vi "DSF.Engine.BuilderManager.Builder FIFO.Write.vi"(8 "error in (no error)":errorcluster, 9 "timeout in ms (0)":i32, 10 "Builder ID":i32, 11 "Builder Manager in":refnum<class "DSF.Engine.BuilderManager.lvclass">) -> (0 "error out":errorcluster, 1 "timed out?":bool, 3 "Builder Manager out":refnum<class "DSF.Engine.BuilderManager.lvclass">)   [LabVIEW 2016, in "DSF.Engine.lvlib" / "DSF.Engine.BuilderManager.lvclass"]
uses:
  DSF.Engine.BuilderManager.lvclass
  DSF.Engine.BuilderManager.lvclass/DSF.Engine.BuilderManager.ctl
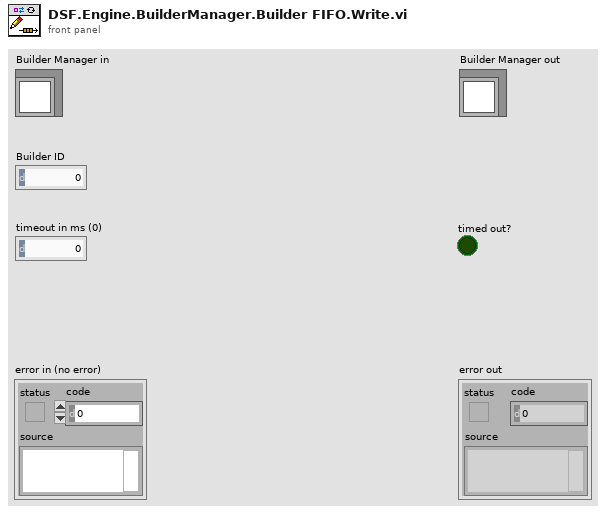
[diagram p1: front panel]
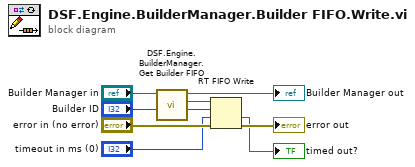
[diagram p0: block diagram]
diagram:
  n1 = call "DSF.Engine.BuilderManager.Get Builder FIFO.vi"("Builder Manager in"="Builder Manager in") -> ("Builder FIFO"=w7:refnum<k33>, "Builder Manager out"=→"Builder Manager out":refnum<class "DSF.Engine.BuilderManager.lvclass">)  [unwired: 9 in]
  n2 = RT FIFO Write(0:w7, 1:"Builder ID", 2:"timeout in ms (0)", 3:"error in (no error)") -> (10:→"timed out?":bool, 11:→"error out":errorcluster)  [unwired: 1 in, 2 out]
